vi "Display Measure Function.vi"(7 "Function (Current)":u16(ring) items=["Current", "Voltage", "Resistance", "Power"], 8 "error in (no error)":errorcluster, 9 "Channel (Channel A)":u16(ring) items=["Channel A", "Channel B"], 10 "Node In":string, 11 "VISA resource name":refnum<visa-resource-name>) -> (0 "error out":errorcluster, 2 "Node Out":string, 3 "VISA resource name out":refnum<visa-resource-name>, 4 "Command String":string)   [LabVIEW 2017, in "Keithley 2600 Series.lvlib"]
doc: "This VI selects the type of measurement to be displayed on the instrument's front panel screen.\n\n<b>Functions and Attributes Used</b>\ndisplay.smuX.measure.func\nX = SMU channel (a or b)"
uses:
  Keithley 2600 Series.lvlib
  Private/GlobalVariables.vi
panel:
  # "(c) 2008 Keithley Instruments, Inc.  ALL RIGHTS RESERVED."
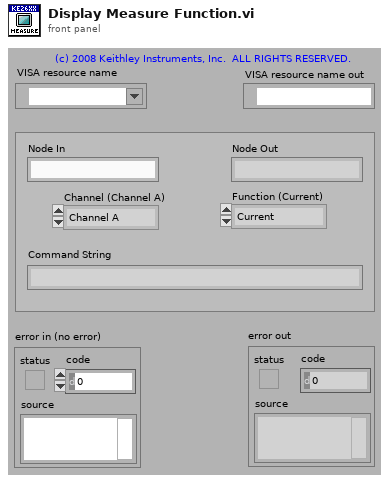
[diagram p1: front panel]
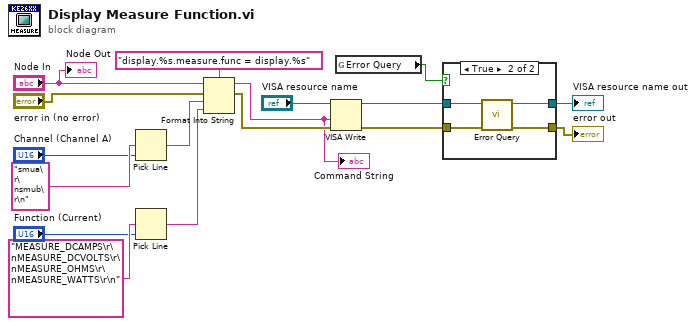
[diagram p0: block diagram]
diagram:
  n1 = Pick Line(multi-line string="smua\r\nsmub\r\n" ("options"), line index="Channel (Channel A)") -> (output string=w6:string)  [unwired: 1 out]
  n2 = Pick Line(multi-line string="MEASURE_DCAMPS\r\nMEASURE_DCVOLTS\r\nMEASURE_OHMS\r\nMEASURE_WATTS\r\n" ("options"), line index="Function (Current)") -> (output string=w5:string)  [unwired: 1 out]
  n3 = Format Into String(format string="display.%s.measure.func = display.%s", initial string="Node In", error in="error in (no error)", w6, w5) -> (resulting string=w1:string, error out=w2:errorcluster)
  "Command String" <- w1
  n4 = VISA Write(VISA resource name="VISA resource name", write buffer=w1, error in (no error)=w2) -> (VISA resource name out=w12:refnum<visa-resource-name>, error out=w11:errorcluster)  [unwired: 1 out]
  n5 = global read "GlobalVariables.vi" "Error Query"() -> (w13:bool)
  n6 = case shown="True" w13 {
    tunnel: w12 -> [w19 w23]
    tunnel: w11 -> [w18 w22]
    tunnel: [w19 w21] -> w9
    tunnel: [w18 w20] -> w10
    frame False {
    }
    frame True {
      n7 = call "Error Query.vi"("error in (no error)"=w22, "VISA resource name"=w23) -> ("error out"=w20:errorcluster, "VISA resource name out"=w21:refnum<visa-resource-name>)  [unwired: 8 out]
    }
  }
  "VISA resource name out" <- w9
  "error out" <- w10
  "Node Out" <- "Node In"
